vi "Write AlicatDev.vi"(8 "error in":errorcluster, 10 "AlicatDev":refnum<class "Alicat.lvclass">[](array[class]), 11 "AlicatCommBank in":refnum<class "AlicatCommBank.lvclass">) -> (0 "error out":errorcluster, 3 "AlicatCommBank out":refnum<class "AlicatCommBank.lvclass">)   [LabVIEW 2015, in "Alicat.lvlib" / "AlicatCommBank.lvclass"]
doc: "Use this accessor to instantiate the different Alicat devices that will be used."
uses:
  AlicatCommBank.lvclass
  Alicat.lvclass
  AlicatCommBank.lvclass/AlicatCommBank.ctl
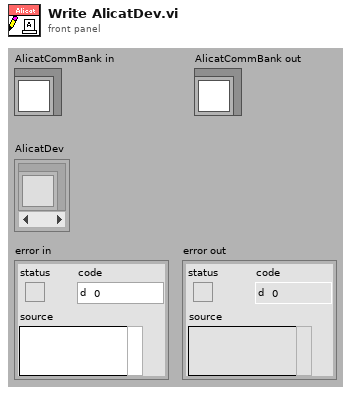
[diagram p1: front panel]
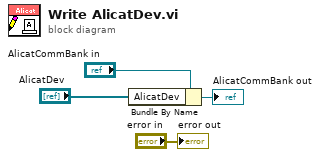
[diagram p0: block diagram]
diagram:
  n1 = Bundle By Name(cluster="AlicatCommBank in", "AlicatDev"="AlicatDev") -> (→"AlicatCommBank out":refnum<class "AlicatCommBank.lvclass">)
  "error out" <- "error in"
